vi "_getKeyList.vi"   [LabVIEW 2022 SP3, in "openDAQ.lvlib" / "daqCoreTypes.lvlib" / "IDict.lvclass"]
uses:
  IDict.lvclass
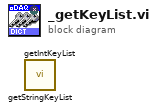
[diagram p0: block diagram]
diagram:
  n1 = call "getStringKeyList.vi"() -> ()  [unwired: 9 in, 3 out]
  n2 = call "getIntKeyList.vi"() -> ()  [unwired: 9 in, 3 out]
